vi "Register Projections.vi"(10 "Projection Info":T1[](array[typedef])) -> ()   [LabVIEW 2013]
doc: "Copyright (c) 2016 Sze Howe Koh\n\nThis Source Code Form is subject to the terms of the Mozilla Public License, v. 2.0. If a copy of the MPL was not distributed with this file, You can obtain one at http://mozilla.org/MPL/2.0/."
uses:
  Data Structures/JSON/Projection Info.ctl
  Param Writers/TypeConv/Action.ctl
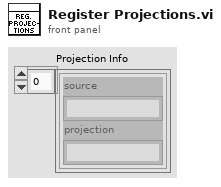
[diagram p1: front panel]
types:
  T1 = typedef "Projection Info.ctl" = cluster{"source":string, "projection":string}
  T2 = typedef "Action.ctl" = enum16{"Register Type", "Register Projection", "Obtain Writer", "Get Projection", "Get Type Path", "Get Type Category"}
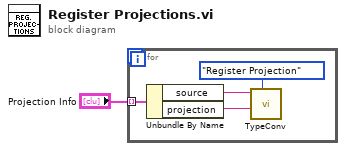
[diagram p0: block diagram]
diagram:
  n1 = for {
    tunnel: "Projection Info" -> [w5] mode=indexing
    n2 = Unbundle By Name(w5) -> ("source"=w3:string, "projection"=w4:string)
    n3 = call "TypeConv.vi"("Action"=Action."Register Projection", "Alternative Name"=w4, "Type Name"=w3) -> ()  [unwired: 4 in, 5 out]
  }
